vi "Child UIDs.vi"(11 "Actor in":refnum<class "Actor.lvclass">) -> (2 "Child UIDs":T1)   [LabVIEW 2025, in "jettl.lvlib" / "Actor.lvlib" / "Actor.lvclass"]
uses:
  Actor.lvclass
  Child UIDs.ctl
  Actor.lvlib
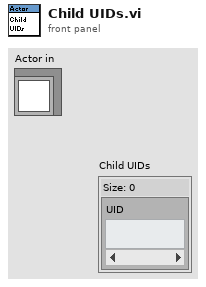
[diagram p1: front panel]
types:
  T1 = typedef "jettl.lvlib/Actor.lvlib/Child UIDs.ctl" = set{string}
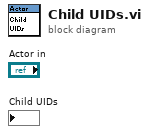
[diagram p0: block diagram]
diagram:
